vi "niRFUtil RFHS Benchmark Stop.vi"(0 "Start Time":u64, 5 "Benchmark Task":T2, 7 "Benchmark Id":T1, 11 "error in (no error)":errorcluster) -> (15 "error out":errorcluster)   [LabVIEW 2015, in "niRFUtil.lvlib"]
uses:
  niRFUtil.lvlib
  niRFUtil RFHS Benchmark Task.ctl
  niRFUtil RFHS Benchmark Id.ctl
  niRFUtil RFHS Util Phases.ctl
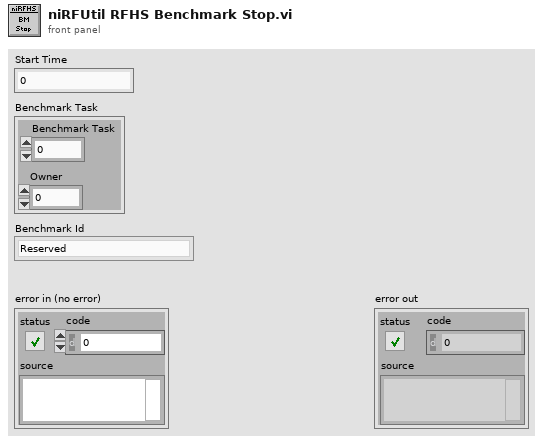
[diagram p1: front panel]
types:
  T1 = typedef "niRFUtil.lvlib/niRFUtil RFHS Benchmark Id.ctl" = enum32{"Reserved", "Gen CRC", "Gen Segment TB", "Gen Turbo Coder", "Gen Rate Matching", "Gen UL Chan Interleaver", "Gen Scramble", "Gen Group Bits", "Gen Modulator", "Gen UL Preconditioning", "Gen Freq2Time", "Gen UL DMRS", "Ana Time2Freq", "Ana EQ", "Ana UL Preconditioning", "Ana Demodulator", "Ana Descrambler", "Ana UL Chan Deinterleaver", "Ana UL HARQ", "Ana AFEM", "Ana Turbo Decoder", "Ana CRC", "TD Perm", "TD Convert AB", "TD Primes", "TD PInv", "TD Alpha", "TD Beta", "TD La", "TD Gamma", "Ana AFEM SF Sync", "Ana Loop"}
  T2 = typedef "niRFUtil.lvlib/niRFUtil RFHS Benchmark Task.ctl" = cluster{"Benchmark Task":u64, "Owner":u32}
  T3 = typedef "niRFUtil.lvlib/niRFUtil RFHS Util Phases.ctl" = enum32{"Reserved", "CreateBenchmarkTask", "CRC", "UE UL Segment Transport Block", "UE UL Read Buffer", "UE UL TC", "UE UL RM", "UE UL CI", "Scramble", "Group Bits", "Benchmark Task Start", "Benchmark Task Stop", "Descramble", "Deinterleave", "eNB UL HARQ", "eNB UL Read Buffer", "eNB UL AFEM", "eNB UL Turbo Decoder", "Get Benchmark Task Data", "G31", "UL Gen Freq2Time", "Gen Power Spectrum", "UL Ana Time2Freq", "Benchmark Task Enter", "Benchmark Task Leave"}
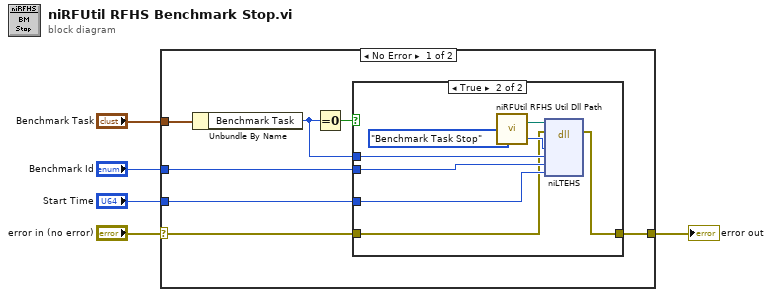
[diagram p0: block diagram]
diagram:
  n1 = case shown="No Error" "error in (no error)" {
    selector: "error in (no error)" -> [w7 w21]
    tunnel: "Benchmark Task" -> [w9 _]
    tunnel: "Benchmark Id" -> [w12 _]
    tunnel: "Start Time" -> [w11 _]
    tunnel: [w6 w21] -> w1
    frame No Error {
      n2 = Unbundle By Name(w9) -> ("Benchmark Task"=w8:u64)
      n3 = Equal To 0?(x=w8) -> (x = 0?=w10:bool)
      n4 = case shown="True" w10 {
        tunnel: w8 -> [_ w18]
        tunnel: w12 -> [_ w17]
        tunnel: w11 -> [_ w16]
        tunnel: w7 -> [w13 w15]
        tunnel: [w13 w14] -> w6
        frame False {
        }
        frame True {
          n5 = call "niRFUtil RFHS Util Dll Path.vi"() -> ("Path"=w20:path)  [unwired: 7 in, 4 out]
          n6 = dll-call lib="C:/ni-rt/system/HPCExecBenchDll.dll" fn="niLTEHS"(path in=w20, error in=w15, "what"=niRFUtil_RFHS_Util_Phases."Benchmark Task Stop" ("Enum"), "benchmarkTask"=w18, "benchId"=w17, "startTime"=w16) -> (error out=w14:errorcluster)  [unwired: 6 in, 1 out]
        }
      }
    }
    frame Error {
    }
  }
  "error out" <- w1
